vi "Position Parse.vi"(8 "Byte 1":u8 format="%.0x", 9 "Byte 2":u8 format="%.0x", 10 "Byte 3":u8 format="%.0x", 11 "Byte 4":u8 format="%.0x") -> (3 "Position":i32)   [LabVIEW 2014, in "ALPHA5 RS485.lvlib"]
uses:
  ALPHA5 RS485.lvlib
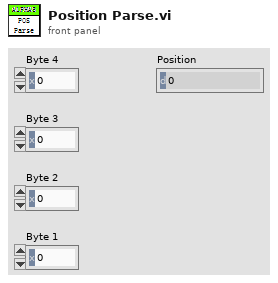
[diagram p1: front panel]
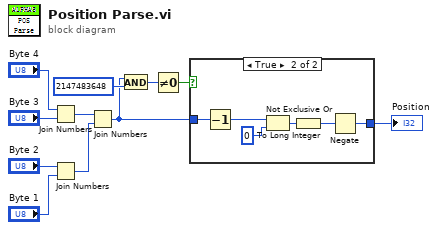
[diagram p0: block diagram]
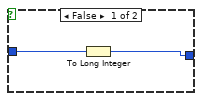
[diagram p2: hidden frame]
diagram:
  n1 = Join Numbers(hi="Byte 4", lo="Byte 3") -> ((hi.lo)=w7:u16)
  n2 = Join Numbers(hi="Byte 2", lo="Byte 1") -> ((hi.lo)=w6:u16)
  n3 = Join Numbers(hi=w7, lo=w6) -> ((hi.lo)=w2:u32)
  n4 = And(x=w2, y=u32 2147483648) -> (x .and. y?=w4:u32)
  n5 = Not Equal To 0?(x=w4) -> (x != 0?=w3:bool)
  n6 = case shown="True" w3 {
    tunnel: w2 -> [w13 w19]
    tunnel: [w12 w14] -> w1
    frame False {
      n7 = To Long Integer(number=w13) -> (32bit integer=w12:i32)
    }
    frame True {
      n8 = Decrement(x=w19) -> (x-1=w18:u32)
      n9 = Not Exclusive Or(1:u32 0 ("y"), 2:w18) -> (0:w16:u32)
      n10 = To Long Integer(number=w16) -> (32bit integer=w15:i32)
      n11 = Negate(x=w15) -> (-x=w14:i32)
    }
  }
  "Position" <- w1
